vi "SailRudderControlLogic.vi"(9 "DesiredHeading":dbl, 10 "NotifierReff":T1, 11 "Commanded Boat Regime":T4) -> (2 "Suggested Rudder Setpoint":T2 min=-0.95 max=0.95 scale=1.0..-1.0, 3 "Suggested Sail Setpoints":T3 {"MainSailSuggestion" min=0.0 max=1.0; "JibSailSuggestion" min=0.0 max=1.0})   [LabVIEW 2013]
doc: "This VI takes in the Commanded Sail Regime and then decides how to set the sails and rudder. The rudder is set with Robot Heading and Desired Heading using an NI-made PID loop. The sails are set up so that they could be controlled each with separate control logic, but currently the boat uses the simple wind-to-sail-lookup-table code to set the sail in almost all cases.\n\nFeb. 2014, Bonnie Ishiguro and Eric Schneider"
uses:
  Data/TypeDefs/Boat Regimes.ctl
  Data/TypeDefs/Sailing Regimes.ctl
  Data/TypeDefs/Emergency Regimes.ctl
  Data/TypeDefs/Sail Set Suggestions.ctl
  Data/TypeDefs/Rudder Set Suggestions.ctl
  Data/TypeDefs/Notifiers.ctl
  Data/TypeDefs/UTM Location.ctl
  Data/TypeDefs/OverrideInformation.ctl
  Data/TypeDefs/OverrideMode.ctl
  Data/TypeDefs/MotorSetup.ctl
  Data/TypeDefs/DynamixelSetupInfo.ctl
  Data/TypeDefs/AirmarStatus.ctl
  Data/TypeDefs/HardwareOnline.ctl
  Data/TypeDefs/DynamixelCycleTracker.ctl
  Utilities/Math/Angles/Angle/Angle.lvclass
panel:
  in  "AbsoluteWindAngle":dbl
  in  "ApparentWindAngle (0-180)":dbl
  in  "Robot Heading":dbl
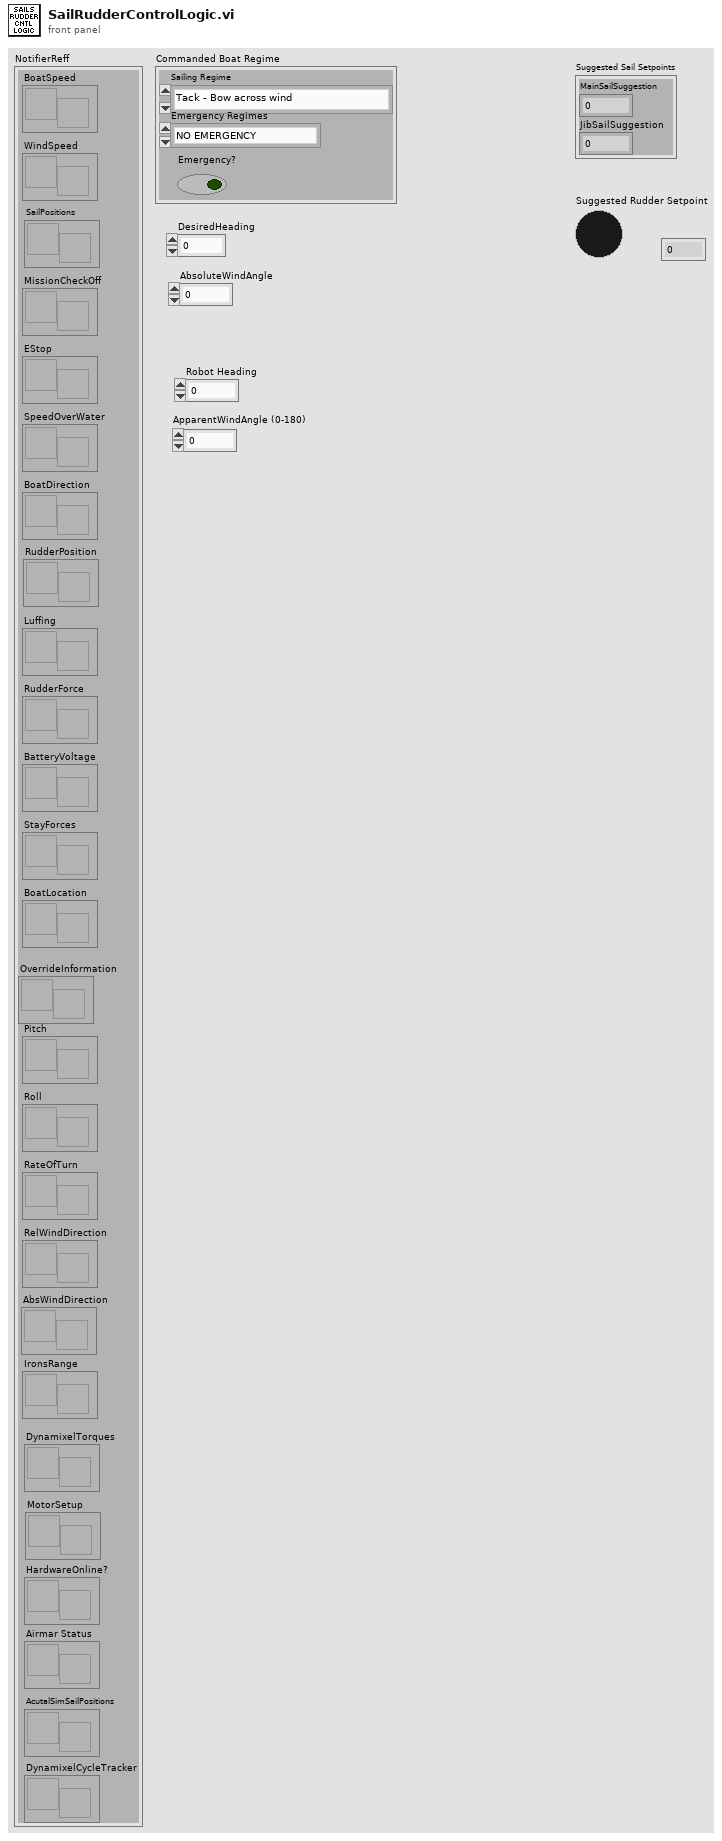
[diagram p1: front panel]
types:
  T1 = typedef "Notifiers.ctl" = cluster{"BoatSpeed":refnum<notifier>, "WindSpeed":refnum<notifier>, "MissionCheckOff":refnum<notifier>, "EStop":refnum<notifier>, "SpeedOverWater":refnum<notifier>, "BoatDirection":refnum<notifier>, "Luffing":refnum<notifier>, "RudderForce":refnum<notifier>, "BatteryVoltage":refnum<notifier>, "StayForces":refnum<notifier>, "BoatLocation":refnum<notifier>, "Pitch":refnum<notifier>, "Roll":refnum<notifier>, "RateOfTurn":refnum<notifier>, "RelWindDirection":refnum<notifier>, "SailPositions":refnum<notifier>, "RudderPosition":refnum<notifier>, "IronsRange":refnum<notifier>, "AbsWindDirection":refnum<notifier>, "OverrideInformation":refnum<notifier>, "DynamixelTorques":refnum<notifier>, "MotorSetup":refnum<notifier>, "Airmar Status":refnum<notifier>, "HardwareOnline?":refnum<notifier>, "AcutalSimSailPositions":refnum<notifier>, "DynamixelCycleTracker":refnum<notifier>}
  T2 = typedef "Rudder Set Suggestions.ctl" = dbl
  T3 = typedef "Sail Set Suggestions.ctl" = cluster{"MainSailSuggestion":dbl, "JibSailSuggestion":dbl}
  T4 = typedef "Boat Regimes.ctl" = cluster{"Sailing Regime":T5, "Emergency Regimes":T6, "Emergency?":bool}
  T5 = typedef "Sailing Regimes.ctl" = enum16{"Tack - Bow across wind", "Upwind - Starboard Tack", "Turn between Upwind/Reach - Starboard Tack", "Reach - Starboard Tack", "Turn between Reach/Run - Starboard Tack", "Run - Starboard Tack", "Jibe - Stern across wind", "Run - Port Tack", "Turn between Reach/Run - Port Tack", "Reach - Port Tack", "Turn between Upwind/Reach - Port Tack", "Upwind - Port Tack"}
  T6 = typedef "Emergency Regimes.ctl" = enum16{"NO EMERGENCY", "No Knockdown", "Obstacle Avoid"}
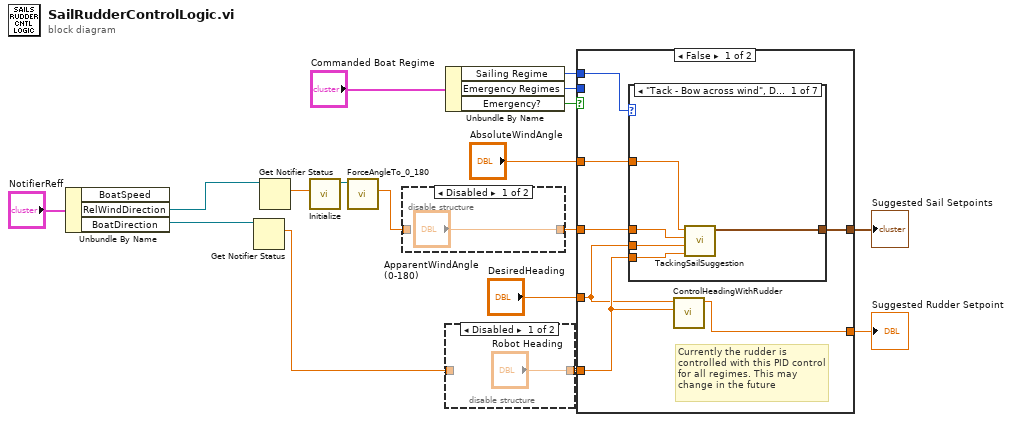
[diagram p0: block diagram]
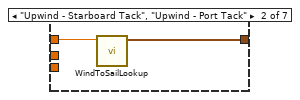
[diagram p4: hidden frame]
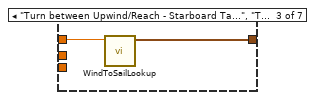
[diagram p5: hidden frame]
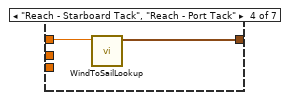
[diagram p6: hidden frame]
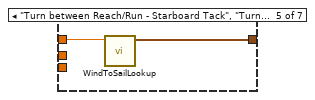
[diagram p7: hidden frame]
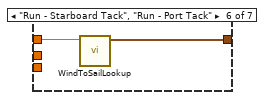
[diagram p8: hidden frame]
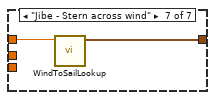
[diagram p9: hidden frame]
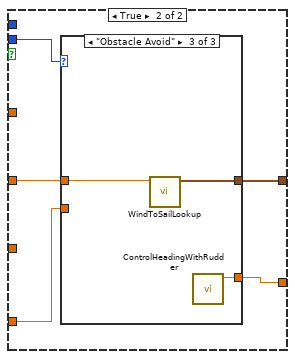
[diagram p10: hidden frame]
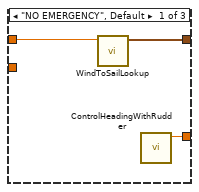
[diagram p11: hidden frame]
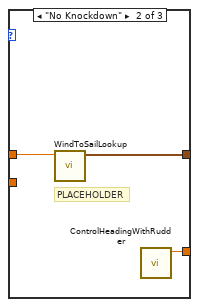
[diagram p12: hidden frame]
diagram:
  n1 = Unbundle By Name("NotifierReff") -> ("RelWindDirection"=w4:refnum<notifier>, "BoatDirection"=w6:refnum<notifier>)  [unwired: 1 out]
  n2 = Get Notifier Status(notifier=w6) -> (current notification=w5:dbl)  [unwired: 1 in, 4 out]
  n3 = Get Notifier Status(notifier=w4) -> (current notification=w3:dbl)  [unwired: 1 in, 4 out]
  n4 = call "Initialize.vi"("Input Angle (Deg.)"=w3) -> ("Angle out"=w2:refnum<class "Angle.lvclass">)  [unwired: 9 in, 1 out]
  n5 = call "ForceAngleTo_0_180.vi"("Angle in"=w2) -> ("Angle out"=w1:dbl)  [unwired: 9 in, 1 out]
  n6 = disable-structure shown="Disabled" {
    disable-tunnel: ["ApparentWindAngle (0-180)" w19] -> w14
    disable-tunnel: w1 -> [_ w19]
    frame Disabled {
    }
    frame Enabled {
    }
  }
  n7 = Unbundle By Name("Commanded Boat Regime") -> ("Sailing Regime"=w16:T5, "Emergency Regimes"=w13:T6, "Emergency?"=w17:bool)
  n8 = disable-structure shown="Disabled" {
    disable-tunnel: ["Robot Heading" w21] -> w10
    disable-tunnel: w5 -> [_ w21]
    frame Disabled {
    }
    frame Enabled {
    }
  }
  n9 = case shown="False" w17 {
    tunnel: w16 -> [w28 _]
    tunnel: w10 -> [w23 w47]
    tunnel: w14 -> [w27 w49]
    tunnel: [w26 w48] -> w12
    tunnel: [w24 w46] -> w11
    tunnel: w13 -> [_ w50]
    tunnel: "AbsoluteWindAngle" -> [w25 _]
    tunnel: "DesiredHeading" -> [w22 _]
    frame False {
      # "Currently the rudder is controlled with this PID control for all regimes. This may change in the future"
      n10 = case shown="\"Tack - Bow across wind\", Default" w28 {
        tunnel: w27 -> [w30 w35 w37 w39 w41 w43 w45]
        tunnel: [w33 w34 w36 w38 w40 w42 w44] -> w26
        tunnel: w25 -> [w32 _ _ _ _ _ _]
        tunnel: w23 -> [w29 _ _ _ _ _ _]
        tunnel: w22 -> [w31 _ _ _ _ _ _]
        frame "Tack - Bow across wind", Default {
          n11 = call "TackingSailSuggestion.vi"("RobotHeading"=w29, "DesiredHeading"=w31, "ApparentWindAngle"=w30, "AbsoluteWindAngle"=w32) -> ("Suggested Sail Setpoints"=w33:T3)  [unwired: 7 in]
        }
        frame "Upwind - Starboard Tack", "Upwind - Port Tack" {
          n12 = call "WindToSailLookup.vi"("ApparentWindAngle"=w35) -> ("Suggested Sail Setpoints"=w34:T3)  [unwired: 10 in]
        }
        frame "Turn between Upwind/Reach - Starboard Tack", "Turn between Upwind/Reach - Port Tack" {
          n13 = call "WindToSailLookup.vi"("ApparentWindAngle"=w37) -> ("Suggested Sail Setpoints"=w36:T3)  [unwired: 10 in]
        }
        frame "Reach - Starboard Tack", "Reach - Port Tack" {
          n14 = call "WindToSailLookup.vi"("ApparentWindAngle"=w39) -> ("Suggested Sail Setpoints"=w38:T3)  [unwired: 10 in]
        }
        frame "Turn between Reach/Run - Starboard Tack", "Turn between Reach/Run - Port Tack" {
          n15 = call "WindToSailLookup.vi"("ApparentWindAngle"=w41) -> ("Suggested Sail Setpoints"=w40:T3)  [unwired: 10 in]
        }
        frame "Run - Starboard Tack", "Run - Port Tack" {
          n16 = call "WindToSailLookup.vi"("ApparentWindAngle"=w43) -> ("Suggested Sail Setpoints"=w42:T3)  [unwired: 10 in]
        }
        frame "Jibe - Stern across wind" {
          n17 = call "WindToSailLookup.vi"("ApparentWindAngle"=w45) -> ("Suggested Sail Setpoints"=w44:T3)  [unwired: 10 in]
        }
      }
      n18 = call "ControlHeadingWithRudder.vi"("Desired Heading"=w22, "Robot Heading"=w23) -> ("Suggested Rudder Setpoint"=w24:T2)  [unwired: 8 in]
    }
    frame True {
      n19 = case shown="\"Obstacle Avoid\"" w50 {
        tunnel: w49 -> [w53 w56 w57]
        tunnel: [w51 w55 w58] -> w48
        tunnel: w47 -> [_ _ _]
        tunnel: [w52 w54 w59] -> w46
        frame "NO EMERGENCY", Default {
          n20 = call "WindToSailLookup.vi"("ApparentWindAngle"=w53) -> ("Suggested Sail Setpoints"=w51:T3)  [unwired: 10 in]
          n21 = call "ControlHeadingWithRudder.vi"() -> ("Suggested Rudder Setpoint"=w52:T2)  [unwired: 10 in]
        }
        frame "No Knockdown" {
          # "PLACEHOLDER"
          n22 = call "WindToSailLookup.vi"("ApparentWindAngle"=w56) -> ("Suggested Sail Setpoints"=w55:T3)  [unwired: 10 in]
          n23 = call "ControlHeadingWithRudder.vi"() -> ("Suggested Rudder Setpoint"=w54:T2)  [unwired: 10 in]
        }
        frame "Obstacle Avoid" {
          n24 = call "WindToSailLookup.vi"("ApparentWindAngle"=w57) -> ("Suggested Sail Setpoints"=w58:T3)  [unwired: 10 in]
          n25 = call "ControlHeadingWithRudder.vi"() -> ("Suggested Rudder Setpoint"=w59:T2)  [unwired: 10 in]
        }
      }
    }
  }
  "Suggested Sail Setpoints" <- w12
  "Suggested Rudder Setpoint" <- w11
